vi "Set Server Internal UEs.vi"(10 "Server Internal UEs":T1, 11 "OOP Server in":refnum<class "TestServer.lvclass">) -> (3 "OOP Server out":refnum<class "TestServer.lvclass">)   [LabVIEW 2019, in "TestServer.lvlib" / "TestServer.lvclass"]
uses:
  TestServer.lvclass
  typeDefs/Server Internal UEs.ctl
  typeDefs/Server Internal Message.ctl
  TestServer.lvclass/TestServer.ctl
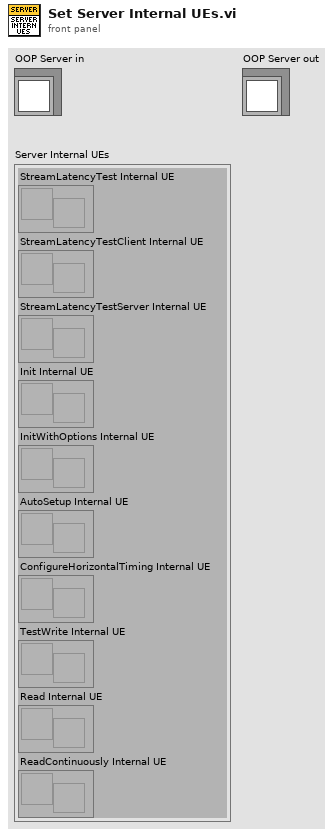
[diagram p1: front panel]
types:
  T1 = typedef "TestServer.lvlib/TestServer.lvclass/Server Internal UEs.ctl" = cluster{"StreamLatencyTest Internal UE":refnum<user-event>, "StreamLatencyTestClient Internal UE":refnum<user-event>, "StreamLatencyTestServer Internal UE":refnum<user-event>, "Init Internal UE":refnum<user-event>, "InitWithOptions Internal UE":refnum<user-event>, "AutoSetup Internal UE":refnum<user-event>, "ConfigureHorizontalTiming Internal UE":refnum<user-event>, "TestWrite Internal UE":refnum<user-event>, "Read Internal UE":refnum<user-event>, "ReadContinuously Internal UE":refnum<user-event>}
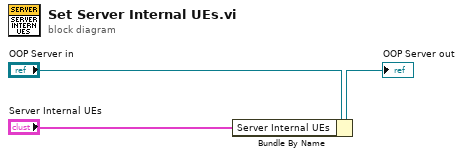
[diagram p0: block diagram]
diagram:
  n1 = Bundle By Name(cluster="OOP Server in", "Server Internal UEs"="Server Internal UEs") -> (→"OOP Server out":refnum<class "TestServer.lvclass">)
